vi "Hide ScrollBars.vi"(8 "error in":errorcluster, 11 "VI Ref in":refnum<vi>) -> (0 "error out":errorcluster, 3 "VI Ref Out":refnum<vi>)   [LabVIEW 2012]
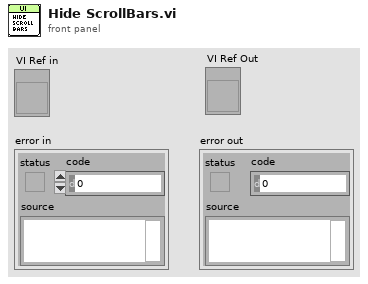
[diagram p1: front panel]
types:
  T1 = enum16{"Always On", "Always Off", "Off While Running"}
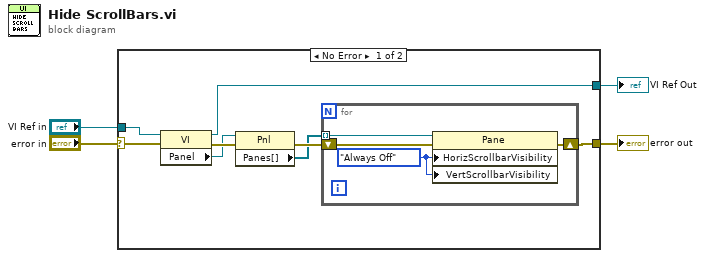
[diagram p0: block diagram]
diagram:
  n1 = case shown="No Error" "error in" {
    selector: "error in" -> [w7 w17]
    tunnel: "VI Ref in" -> [w6 _]
    tunnel: [w12 w17] -> w3
    tunnel: [w5 _] -> w1
    frame No Error {
      n2 = property class="VI"(reference=w6, error in=w7) -> (reference out=w5:refnum<vi>, error out=w9:errorcluster, "Panel"=w8:refnum<vi>)
      n3 = property class="Pnl"(reference=w8, error in=w9) -> (error out=w11:errorcluster, "Panes[]"=w10:refnum<vi>[])  [unwired: 1 out]
      n4 = for {
        tunnel: w10 -> [w16] mode=indexing
        shift-right: [w14] -> w12
        shift-left: w11 -> [w15]
        w13 = T1."Always Off" ("Horizontal Scrollbar Visibility")
        n5 = property class="Pane"(reference=w16, error in=w15, "HorizScrollbarVisibility"=w13, "VertScrollbarVisibility"=w13) -> (error out=w14:errorcluster)  [unwired: 1 out]
      }
    }
    frame Error {
    }
  }
  "error out" <- w3
  "VI Ref Out" <- w1
